vi "Variant to String.vi"(11 "Variant":variant) -> (2 "error out":errorcluster, 3 "String":string)   [LabVIEW 2020, in "Vecto.lvlib" / "StringGroup.lvclass"]
uses:
  StringGroup.lvclass
  StringGroup.lvclass/StringGroup.ctl
  <vilib>/Utility/Data Type/NI_Data Type.lvlib
  lv-web-crypto/lv-json/JSON/JSON.lvlib
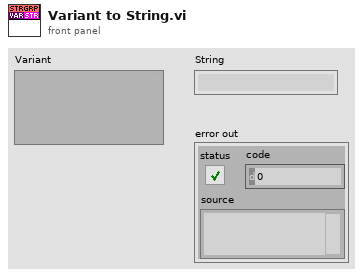
[diagram p1: front panel]
types:
  T1 = typedef "NI_Data Type.lvlib/Data Type.ctl" = enum8{"Invalid Type", "Void", "I8", "I16", "I32", "I64", "U8", "U16", "U32", "U64", "Single Float", "Double Float", "Extended Float", "Single Complex", "Double Complex", "Extended Complex", "Enum U8", "Enum U16", "Enum U32", "Enum U64", "Single Float With Unit", "Double Float With Unit", "Extended Float With Unit", "Single Complex with Unit", "Double Complex with Unit", "Extended Complex with Unit", "Boolean", "String", "Path", "Picture", "Tag", "Array", "Cluster", "Variant", "LV Variant", "Waveform", "Timestamp", "Digital Waveform", "Digital Data", "ExpressData", "Refnum", "External Data", "VI", "Poly VI", "LabVIEW Class Instance", "Fixed Point", "Set Collection", "Map Collection"}
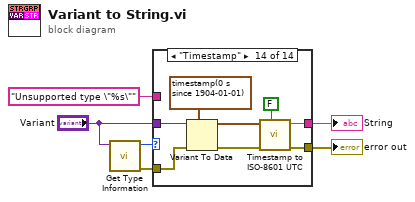
[diagram p0: block diagram]
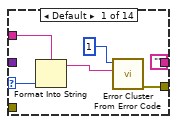
[diagram p2: hidden frame]
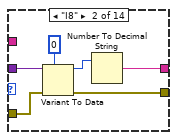
[diagram p3: hidden frame]
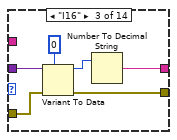
[diagram p4: hidden frame]
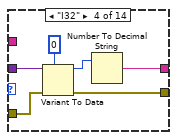
[diagram p5: hidden frame]
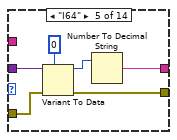
[diagram p6: hidden frame]
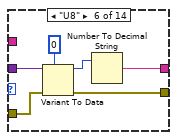
[diagram p7: hidden frame]
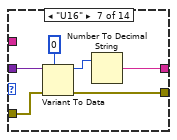
[diagram p8: hidden frame]
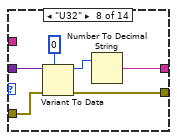
[diagram p9: hidden frame]
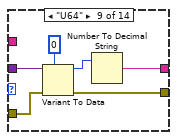
[diagram p10: hidden frame]
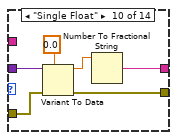
[diagram p11: hidden frame]
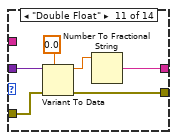
[diagram p12: hidden frame]
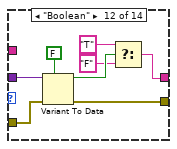
[diagram p13: hidden frame]
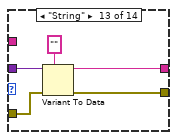
[diagram p14: hidden frame]
diagram:
  n1 = call <vilib>:"Get Type Information.vi"("variant"="Variant") -> ("error out"=w4:errorcluster, "type"=w6:T1)  [unwired: 6 in, 3 out]
  n2 = case shown="\"Timestamp\"" w6 {
    selector: w6 -> [w9 _ _ _ _ _ _ _ _ _ _ _ _ _]
    tunnel: "Variant" -> [_ w18 w24 w30 w36 w42 w48 w54 w60 w66 w72 w80 w85 w92]
    tunnel: w4 -> [_ w16 w22 w28 w34 w40 w46 w52 w58 w64 w70 w78 w83 w91]
    tunnel: [w11 w15 w21 w27 w33 w39 w45 w51 w57 w63 w69 w77 w82 w90] -> w2
    tunnel: ["" w13 w19 w25 w31 w37 w43 w49 w55 w61 w67 w73 w81 w88] -> w3
    tunnel: "Unsupported type \"%s\"" -> [w7 _ _ _ _ _ _ _ _ _ _ _ _ _]
    frame Default {
      n3 = Format Into String(format string=w7, w9) -> (resulting string=w8:string)  [unwired: 2 in, 1 out]
      n4 = call <vilib>:"Error Cluster From Error Code.vi"("error message (\"\")"=w8, "error code (0)"=1) -> ("error out"=w11:errorcluster)  [unwired: 7 in]
    }
    frame "I8" {
      n5 = Variant To Data(error in=w16, type=i8 0, Variant=w18) -> (data=w14:i8, error out=w15:errorcluster)
      n6 = Number To Decimal String(number=w14) -> (decimal integer string=w13:string)  [unwired: 1 in]
    }
    frame "I16" {
      n7 = Variant To Data(error in=w22, type=i16 0, Variant=w24) -> (data=w20:i16, error out=w21:errorcluster)
      n8 = Number To Decimal String(number=w20) -> (decimal integer string=w19:string)  [unwired: 1 in]
    }
    frame "I32" {
      n9 = Variant To Data(error in=w28, type=0, Variant=w30) -> (data=w26:i32, error out=w27:errorcluster)
      n10 = Number To Decimal String(number=w26) -> (decimal integer string=w25:string)  [unwired: 1 in]
    }
    frame "I64" {
      n11 = Variant To Data(error in=w34, type=i64 0, Variant=w36) -> (data=w32:i64, error out=w33:errorcluster)
      n12 = Number To Decimal String(number=w32) -> (decimal integer string=w31:string)  [unwired: 1 in]
    }
    frame "U8" {
      n13 = Variant To Data(error in=w40, type=u8 0, Variant=w42) -> (data=w38:u8, error out=w39:errorcluster)
      n14 = Number To Decimal String(number=w38) -> (decimal integer string=w37:string)  [unwired: 1 in]
    }
    frame "U16" {
      n15 = Variant To Data(error in=w46, type=u16 0, Variant=w48) -> (data=w44:u16, error out=w45:errorcluster)
      n16 = Number To Decimal String(number=w44) -> (decimal integer string=w43:string)  [unwired: 1 in]
    }
    frame "U32" {
      n17 = Variant To Data(error in=w52, type=u32 0, Variant=w54) -> (data=w50:u32, error out=w51:errorcluster)
      n18 = Number To Decimal String(number=w50) -> (decimal integer string=w49:string)  [unwired: 1 in]
    }
    frame "U64" {
      n19 = Variant To Data(error in=w58, type=u64 0, Variant=w60) -> (data=w56:u64, error out=w57:errorcluster)
      n20 = Number To Decimal String(number=w56) -> (decimal integer string=w55:string)  [unwired: 1 in]
    }
    frame "Single Float" {
      n21 = Variant To Data(error in=w64, type=sgl 0.0, Variant=w66) -> (data=w62:sgl, error out=w63:errorcluster)
      n22 = Number To Fractional String(number=w62) -> (F-format string=w61:string)  [unwired: 3 in]
    }
    frame "Double Float" {
      n23 = Variant To Data(error in=w70, type=0.0, Variant=w72) -> (data=w68:dbl, error out=w69:errorcluster)
      n24 = Number To Fractional String(number=w68) -> (F-format string=w67:string)  [unwired: 3 in]
    }
    frame "Boolean" {
      n25 = Variant To Data(error in=w78, type=FALSE, Variant=w80) -> (data=w76:bool, error out=w77:errorcluster)
      n26 = Select(t="T", s=w76, f="F") -> (s? t:f=w73:string)
    }
    frame "String" {
      n27 = Variant To Data(error in=w83, type="", Variant=w85) -> (data=w81:string, error out=w82:errorcluster)
    }
    frame "Timestamp" {
      n28 = Variant To Data(error in=w91, type=timestamp(0 s since 1904-01-01), Variant=w92) -> (data=w89:timestamp, error out=w90:errorcluster)
      n29 = call "Timestamp to ISO-8601 UTC.vi"("Now for Unset? (T)"=FALSE, "Time Stamp"=w89) -> ("ISO 8601 UTC"=w88:string)  [unwired: 9 in]
    }
  }
  "String" <- w3
  "error out" <- w2
